vi "IMS Stepper Wait for Move.vi"(0 "Instrument Address":refnum<visa-resource-name>, 1 "Motor Number":u32=1 min=1 max=255 step=1, 3 "error in (no error)":errorcluster) -> (5 "error out":errorcluster)   [LabVIEW 2018]
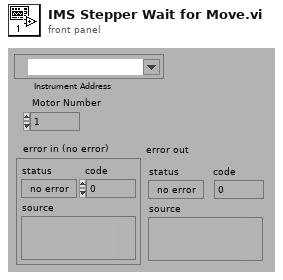
[diagram p1: front panel]
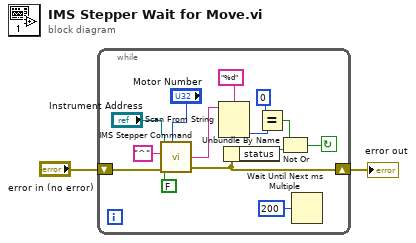
[diagram p0: block diagram]
diagram:
  n1 = while {
    shift-left: "error in (no error)" -> [w12]
    shift-right: [w11] -> w1
    stop <- w10 continue-if-true
    n2 = call "IMS Stepper Command.vi"("Instrument Address"="Instrument Address", "Motor Number"="Motor Number", "Command"="^", "Mode"=FALSE, "error in (no error)"=w12) -> ("Response"=w5:string, "error out"=w11:errorcluster)  [unwired: 1 in, 1 out]
    n3 = Scan From String(format string="%d", input string=w5) -> (output 1=w6:i32)  [unwired: 3 in, 3 out]
    n4 = Unbundle By Name(w11) -> ("status"=w9:bool)
    n5 = Equal?(x=0, y=w6) -> (x = y?=w8:bool)
    n6 = Not Or(1:w9, 2:w8) -> (0:w10:bool)
    n7 = Wait Until Next ms Multiple(millisecond multiple=u32 200) -> ()  [unwired: 1 out]
  }
  "error out" <- w1
